vi "Next Value (NT).vi"(8 "error in (no error)":errorcluster, 9 "timeout":dbl[unit]=1.0, 10 "default value":refnum<class "NT Base.lvclass">, 11 "Subscription in":refnum<class "Subscription.lvclass">) -> (0 "error out":errorcluster, 1 "timed out?":bool, 2 "value":refnum<class "NT Base.lvclass">, 3 "Subscription out":refnum<class "Subscription.lvclass">, 5 "PV name":string)   [LabVIEW 2020, in "PV Access.lvlib" / "PVA Client.lvlib" / "Subscription.lvclass"]
uses:
  Subscription.lvclass
  PV Data/NT Base/NT Base.lvclass
  Subscription.lvclass/Subscription.ctl
  PV Data/PV Data/PV Data.lvclass
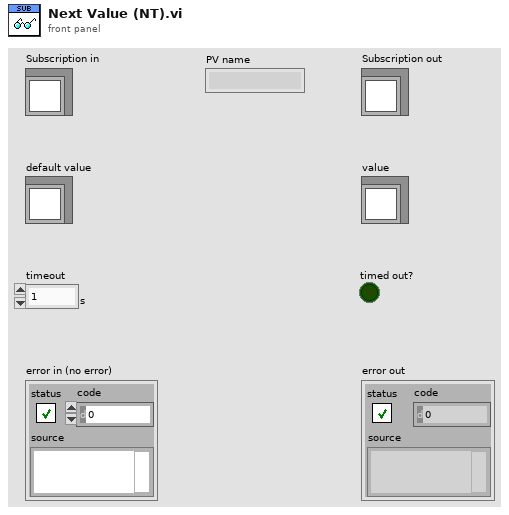
[diagram p1: front panel]
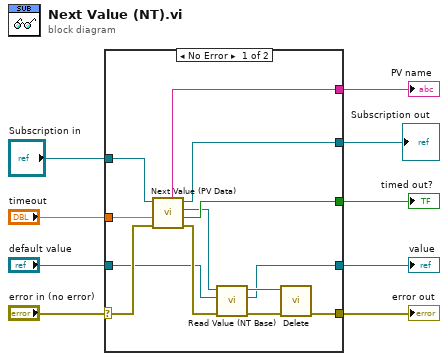
[diagram p0: block diagram]
diagram:
  n1 = case shown="No Error" "error in (no error)" {
    selector: "error in (no error)" -> [w20 w25]
    tunnel: [w10 w25] -> w8
    tunnel: [w21 w24] -> w6
    tunnel: "Subscription in" -> [w22 w24]
    tunnel: "timeout" -> [w19 _]
    tunnel: "default value" -> [w13 w23]
    tunnel: [w11 w23] -> w1
    tunnel: [w18 _] -> w3
    tunnel: [w17 _] -> w2
    frame No Error {
      n2 = call "Next Value (PV Data).vi"("error in (no error)"=w20, "timeout"=w19, "Subscription in"=w22) -> ("error out"=w16:errorcluster, "timed out?"=w18:bool, "PV Data"=w12:refnum<class "PV Data.lvclass">, "Subscription out"=w21:refnum<class "Subscription.lvclass">, "PV name"=w17:string)  [unwired: 4 in]
      n3 = call "Read Value (NT Base).vi"("error in (no error)"=w16, "default value"=w13, "PV Data in"=w12) -> ("error out"=w15:errorcluster, "value"=w11:refnum<class "NT Base.lvclass">, "PV Data out"=w14:refnum<class "PV Data.lvclass">)  [unwired: 6 in]
      n4 = call "Delete.vi"("error in (no error)"=w15, "PV Data in"=w14) -> ("error out"=w10:errorcluster)  [unwired: 9 in]
    }
    frame Error {
    }
  }
  "error out" <- w8
  "Subscription out" <- w6
  "value" <- w1
  "timed out?" <- w3
  "PV name" <- w2
